vi "Process CAN Data.vi"(5 "Pause":bool, 7 "Init?":bool, 8 "error in (no error)":errorcluster, 9 "Timed Out?":bool, 10 "Sort By ID":bool, 11 "CAN Frames (from XNET Read)":T1[](array[typedef]) {"payload" format="%x"; "timestamp" format="%<%.7X\n%x>T"; "type" items=["CAN Data"=0, "CAN Remote"=1, "CAN Bus Error"=2, "CAN 2.0 Data"=8, "CAN FD Data"=16, "CAN FD+BRS Data"=24, "J1939 Data"=192, "Delay"=224, "Log Trigger"=225, "Start Trigger"=226]; "identifier" format="%x"}) -> (0 "error out":errorcluster, 3 "Output Array":string[][](array[string]))   [LabVIEW 2019, in "CAN Streaming Support Workspace Shared.lvlib"]
uses:
  CAN Streaming Support Workspace Shared.lvlib
  <vilib>/xnet/xnet.llb/XNET Frame CAN.ctl
  <vilib>/xnet/xnet.llb/XNET Frame Type CAN.ctl
  <userlib>/_OpenG.lib/array/array.llb/Sort 2D Array (String)__ogtk.vi
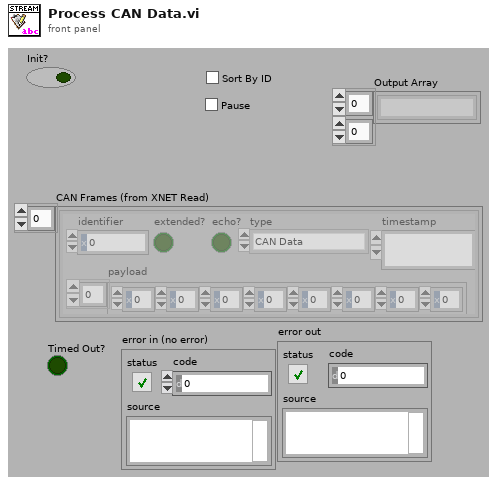
[diagram p1: front panel]
types:
  T1 = typedef "XNET Frame CAN.ctl" = cluster{"timestamp":timestamp, "payload":u8[], "identifier":u32, "type":T2, "extended?":bool, "echo?":bool}
  T2 = typedef "XNET Frame Type CAN.ctl" = u8
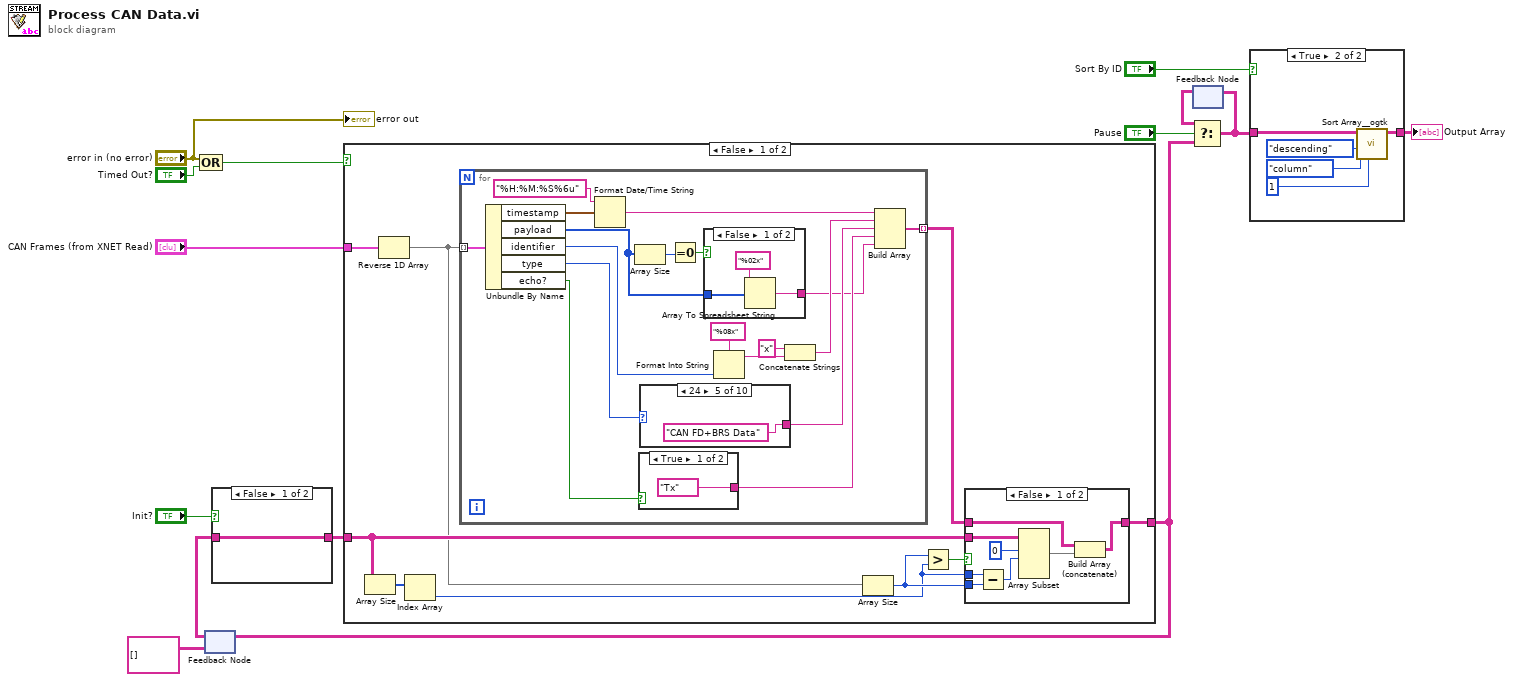
[diagram p0: block diagram]
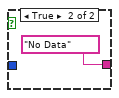
[diagram p3: hidden frame]
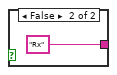
[diagram p4: hidden frame]
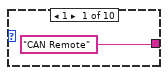
[diagram p5: hidden frame]
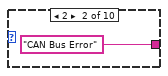
[diagram p6: hidden frame]
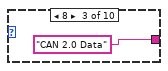
[diagram p7: hidden frame]
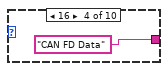
[diagram p8: hidden frame]
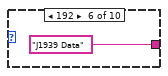
[diagram p9: hidden frame]
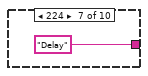
[diagram p10: hidden frame]
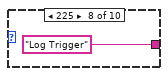
[diagram p11: hidden frame]
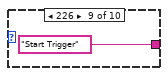
[diagram p12: hidden frame]
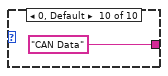
[diagram p13: hidden frame]
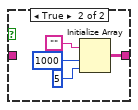
[diagram p15: hidden frame]
diagram:
  n1 = Compound Arithmetic op=OR("error in (no error)", "Timed Out?") -> (w4:bool)
  n2 = feedback #1(string[][] [] ("Sorted Array out")) -> (w11:string[][])
  n3 = case shown="False" "Init?" {
    tunnel: [w15 w17] -> w12
    tunnel: w11 -> [w15 _]
    frame False {
    }
    frame True {
      n4 = Initialize Array("", 1000 ("dimension size"), 5 ("Dimension Size")) -> (w17:string[][])
    }
  }
  n5 = case shown="False" w4 {
    tunnel: "CAN Frames (from XNET Read)" -> [w26 _]
    tunnel: w12 -> [w23 w72]
    tunnel: [w24 w72] -> w8
    frame False {
      n6 = Array Size(array=w23) -> (size(s)=w22:i32[])
      n7 = Reverse 1D Array(array=w26) -> (reversed array=w20:T1[])
      n8 = Index Array(array=w22) -> (element=w21:i32)  [unwired: 1 in]
      n9 = for {
        tunnel: w20 -> [w55] mode=indexing
        tunnel: [w38] -> w27 mode=indexing
        n10 = Unbundle By Name(w55) -> ("timestamp"=w54:timestamp, "payload"=w47:u8[], "identifier"=w53:u32, "type"=w52:T2, "echo?"=w50:bool)
        n11 = Format Date/Time String(time format string (%c)="%H:%M:%S%6u", seconds (now)=w54) -> (date/time string=w40:string)  [unwired: 1 in]
        n12 = Array Size(array=w47) -> (size(s)=w49:i32)
        n13 = case shown="True" w50 {
          tunnel: ["Tx" "Rx"] -> w46
          frame True {
          }
          frame False {
          }
        }
        n14 = case shown="24" w52 {
          tunnel: ["CAN Remote" "CAN Bus Error" "CAN 2.0 Data" "CAN FD Data" "CAN FD+BRS Data" "J1939 Data" "Delay" "Log Trigger" "Start Trigger" "CAN Data"] -> w51
          frame 1 {
          }
          frame 2 {
          }
          frame 8 {
          }
          frame 16 {
          }
          frame 24 {
          }
          frame 192 {
          }
          frame 224 {
          }
          frame 225 {
          }
          frame 226 {
          }
          frame 0, Default {
          }
        }
        n15 = Equal To 0?(x=w49) -> (x = 0?=w48:bool)
        n16 = case shown="False" w48 {
          tunnel: [w57 "No Data"] -> w39
          tunnel: w47 -> [w58 _]
          frame False {
            n17 = Array To Spreadsheet String(array=w58, 3:"%02x" ("format string")) -> (spreadsheet string=w57:string)  [unwired: 1 in]
          }
          frame True {
          }
        }
        n18 = Format Into String(format string="%08x", w53) -> (resulting string=w43:string)  [unwired: 2 in, 1 out]
        n19 = Concatenate Strings("x" ("string"), w43) -> (w42:string)
        n20 = Build Array(w40, w42, w51, w46, w39) -> (w38:string[])
      }
      n21 = Array Size(array=w20) -> (size(s)=w25:i32)
      n22 = Greater?(x=w25, y=w21) -> (0:w28:bool)
      n23 = case shown="False" w28 {
        tunnel: w27 -> [w30 w37]
        tunnel: w21 -> [w36 _]
        tunnel: [w29 w37] -> w24
        tunnel: w23 -> [w34 _]
        tunnel: w25 -> [w35 _]
        frame False {
          n24 = Subtract(x=w36, y=w35) -> (x-y=w32:i32)
          n25 = Array Subset(array=w34, index (row)=0 ("index"), length (row)=w32) -> (w31:string[][])  [unwired: 2 in]
          n26 = Build Array (concatenate)(w30, w31) -> (w29:string[][])
        }
        frame True {
        }
      }
    }
    frame True {
    }
  }
  n27 = feedback-in #1(w8) -> ()
  n28 = feedback #2() -> (w7:string[][])  [unwired: 1 in]
  n29 = Select(t=w7, s="Pause", f=w8) -> (s? t:f=w1:string[][])
  n30 = feedback-in #2(w1) -> ()
  n31 = case shown="True" "Sort By ID" {
    tunnel: w1 -> [w73 w78]
    tunnel: [w73 w77] -> w2
    frame False {
    }
    frame True {
      n32 = call-poly <userlib>:"Sort Array__ogtk.vi"("Column/Row to Sort By"=u32 1, "Sort By in"=enum16{"row", "column"}."column", "Order"=enum16{"ascending", "descending"}."descending", "Array in"=w78) -> ("Sorted Array out"=w77:string[][])  [unwired: 4 in, 3 out]
    }
  }
  "Output Array" <- w2
  "error out" <- "error in (no error)"
